vi "Rotations.vi"() -> (3 "Rotations":cluster{"Rotation":T1}[](array[cluster])=[{"Rotation"=[[1.0, 0.0, 0.0], [0.0, 1.0, 0.0], [0.0, 0.0, 1.0]]}, {"Rotation"=[[1.0, 0.0, 0.0], [0.0, 0.0, -1.0], [0.0, 1.0, 0.0]]}, {"Rotation"=[[1.0, 0.0, 0.0], [0.0, -1.0, 0.0], [0.0, 0.0, -1.0]]}, {"Rotation"=[[1.0, 0.0, 0.0], [0.0, 0.0, 1.0], [0.0, -1.0, 0.0]]}, {"Rotation"=[[0.0, -1.0, 0.0], [1.0, 0.0, 0.0], [0.0, 0.0, 1.0]]}, {"Rotation"=[[0.0, 0.0, 1.0], [1.0, 0.0, 0.0], [0.0, 1.0, 0.0]]}, {"Rotation"=[[0.0, 1.0, 0.0], [1.0, 0.0, 0.0], [0.0, 0.0, -1.0]]}, {"Rotation"=[[0.0, 0.0, -1.0], [1.0, 0.0, 0.0], [0.0, -1.0, 0.0]]}, {"Rotation"=[[-1.0, 0.0, 0.0], [0.0, -1.0, 0.0], [0.0, 0.0, 1.0]]}, {"Rotation"=[[-1.0, 0.0, 0.0], [0.0, 0.0, -1.0], [0.0, -1.0, 0.0]]}, {"Rotation"=[[-1.0, 0.0, 0.0], [0.0, 1.0, 0.0], [0.0, 0.0, -1.0]]}, {"Rotation"=[[-1.0, 0.0, 0.0], [0.0, 0.0, 1.0], [0.0, 1.0, 0.0]]}, {"Rotation"=[[0.0, 1.0, 0.0], [-1.0, 0.0, 0.0], [0.0, 0.0, 1.0]]}, {"Rotation"=[[0.0, 0.0, 1.0], [-1.0, 0.0, 0.0], [0.0, -1.0, 0.0]]}, {"Rotation"=[[0.0, -1.0, 0.0], [-1.0, 0.0, 0.0], [0.0, 0.0, -1.0]]}, {"Rotation"=[[0.0, 0.0, -1.0], [-1.0, 0.0, 0.0], [0.0, 1.0, 0.0]]}, {"Rotation"=[[0.0, 0.0, -1.0], [0.0, 1.0, 0.0], [1.0, 0.0, 0.0]]}, {"Rotation"=[[0.0, 1.0, 0.0], [0.0, 0.0, 1.0], [1.0, 0.0, 0.0]]}, {"Rotation"=[[0.0, 0.0, 1.0], [0.0, -1.0, 0.0], [1.0, 0.0, 0.0]]}, {"Rotation"=[[0.0, -1.0, 0.0], [0.0, 0.0, -1.0], [1.0, 0.0, 0.0]]}, {"Rotation"=[[0.0, 0.0, -1.0], [0.0, -1.0, 0.0], [-1.0, 0.0, 0.0]]}, {"Rotation"=[[0.0, -1.0, 0.0], [0.0, 0.0, 1.0], [-1.0, 0.0, 0.0]]}, {"Rotation"=[[0.0, 0.0, 1.0], [0.0, 1.0, 0.0], [-1.0, 0.0, 0.0]]}, {"Rotation"=[[0.0, 1.0, 0.0], [0.0, 0.0, -1.0], [-1.0, 0.0, 0.0]]}])   [LabVIEW 2020]
uses:
  <vilib>/Analysis/Matrix/Datatypes/RealMatrix.ctl
  <vilib>/Analysis/Matrix/NI_Matrix.lvlib
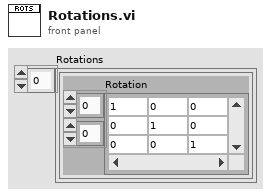
[diagram p1: front panel]
types:
  T1 = typedef "NI_Matrix.lvlib/RealMatrix.ctl" = dbl[][]
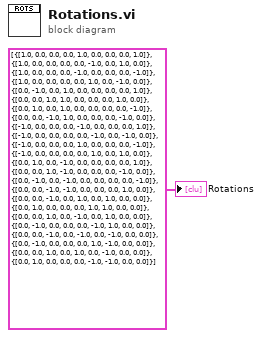
[diagram p0: block diagram]
diagram:
  "Rotations" <- cluster{"Real Matrix":T1}[] [{"Real Matrix"=[[1.0, 0.0, 0.0], [0.0, 1.0, 0.0], [0.0, 0.0, 1.0]]}, {"Real Matrix"=[[1.0, 0.0, 0.0], [0.0, 0.0, -1.0], [0.0, 1.0, 0.0]]}, {"Real Matrix"=[[1.0, 0.0, 0.0], [0.0, -1.0, 0.0], [0.0, 0.0, -1.0]]}, {"Real Matrix"=[[1.0, 0.0, 0.0], [0.0, 0.0, 1.0], [0.0, -1.0, 0.0]]}, {"Real Matrix"=[[0.0, -1.0, 0.0], [1.0, 0.0, 0.0], [0.0, 0.0, 1.0]]}, {"Real Matrix"=[[0.0, 0.0, 1.0], [1.0, 0.0, 0.0], [0.0, 1.0, 0.0]]}, {"Real Matrix"=[[0.0, 1.0, 0.0], [1.0, 0.0, 0.0], [0.0, 0.0, -1.0]]}, {"Real Matrix"=[[0.0, 0.0, -1.0], [1.0, 0.0, 0.0], [0.0, -1.0, 0.0]]}, {"Real Matrix"=[[-1.0, 0.0, 0.0], [0.0, -1.0, 0.0], [0.0, 0.0, 1.0]]}, {"Real Matrix"=[[-1.0, 0.0, 0.0], [0.0, 0.0, -1.0], [0.0, -1.0, 0.0]]}, {"Real Matrix"=[[-1.0, 0.0, 0.0], [0.0, 1.0, 0.0], [0.0, 0.0, -1.0]]}, {"Real Matrix"=[[-1.0, 0.0, 0.0], [0.0, 0.0, 1.0], [0.0, 1.0, 0.0]]}, {"Real Matrix"=[[0.0, 1.0, 0.0], [-1.0, 0.0, 0.0], [0.0, 0.0, 1.0]]}, {"Real Matrix"=[[0.0, 0.0, 1.0], [-1.0, 0.0, 0.0], [0.0, -1.0, 0.0]]}, {"Real Matrix"=[[0.0, -1.0, 0.0], [-1.0, 0.0, 0.0], [0.0, 0.0, -1.0]]}, {"Real Matrix"=[[0.0, 0.0, -1.0], [-1.0, 0.0, 0.0], [0.0, 1.0, 0.0]]}, {"Real Matrix"=[[0.0, 0.0, -1.0], [0.0, 1.0, 0.0], [1.0, 0.0, 0.0]]}, {"Real Matrix"=[[0.0, 1.0, 0.0], [0.0, 0.0, 1.0], [1.0, 0.0, 0.0]]}, {"Real Matrix"=[[0.0, 0.0, 1.0], [0.0, -1.0, 0.0], [1.0, 0.0, 0.0]]}, {"Real Matrix"=[[0.0, -1.0, 0.0], [0.0, 0.0, -1.0], [1.0, 0.0, 0.0]]}, {"Real Matrix"=[[0.0, 0.0, -1.0], [0.0, -1.0, 0.0], [-1.0, 0.0, 0.0]]}, {"Real Matrix"=[[0.0, -1.0, 0.0], [0.0, 0.0, 1.0], [-1.0, 0.0, 0.0]]}, {"Real Matrix"=[[0.0, 0.0, 1.0], [0.0, 1.0, 0.0], [-1.0, 0.0, 0.0]]}, {"Real Matrix"=[[0.0, 1.0, 0.0], [0.0, 0.0, -1.0], [-1.0, 0.0, 0.0]]}]
